vi "Shooter Immediate.vi"(7 "Description":string, 8 "Command Info In":T1, 9 "Deadband Value":dbl=0.01, 10 "LimeLightDistance?":bool, 11 "Setpoint":dbl) -> (0 "Command Info Out":T1)   [LabVIEW 2019]
doc: "This template includes code for deadband comparision to avoid excessive command scheduling. It is particularly useful for joystick-driven commands.\n\nBe sure to right-click and select New from Template and save with a new command name."
uses:
  <vilib>/Rock Robotics/WPI/Framework/Command Status Info.ctl
  <vilib>/Rock Robotics/WPI/Framework/Completion Status.ctl
  <vilib>/Rock Robotics/WPI/Framework/Completion Notifier.ctl
  Implementation/Shooter Setpoints.ctl
  Implementation/Shooter Operations.ctl
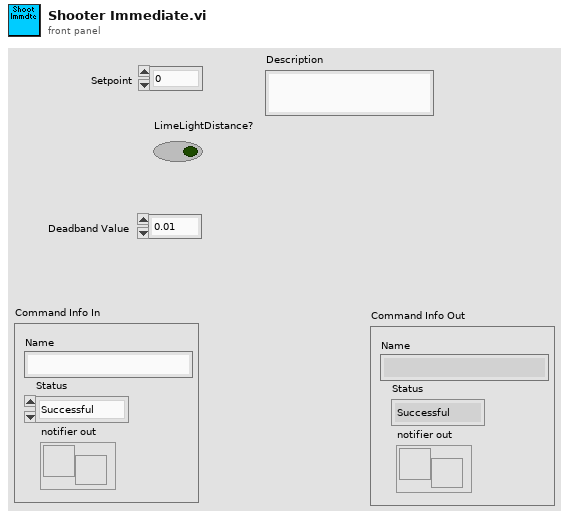
[diagram p1: front panel]
types:
  T1 = typedef "Command Status Info.ctl" = cluster{"Name":string, "Status":T2, "notifier out":T3}
  T2 = typedef "Completion Status.ctl" = enum16{"Successful", "Aborted", "Incomplete"}
  T3 = typedef "Completion Notifier.ctl" = refnum<notifier>
  T4 = typedef "Shooter Setpoints.ctl" = cluster{"Operation":T5, "Setpoint":dbl, "Duration":dbl, "LimelightSpeed":bool}
  T5 = typedef "Shooter Operations.ctl" = enum16{"Reserve", "Read Current", "Immediate", "Shoot for Time"}
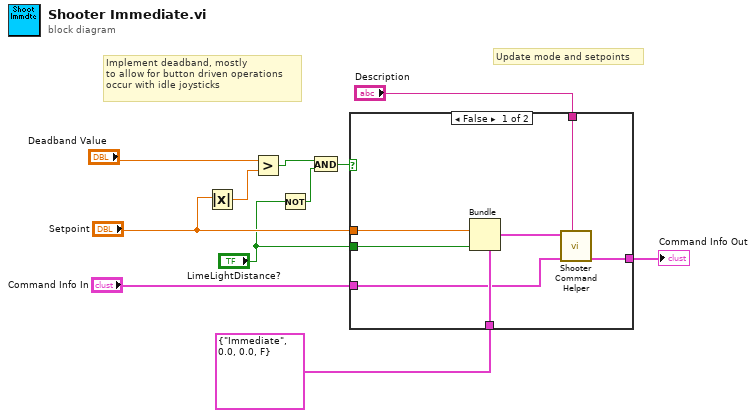
[diagram p0: block diagram]
diagram:
  # "Implement deadband, mostly\nto allow for button driven operations\noccur with idle joysticks"
  # "Update mode and setpoints"
  n1 = Absolute Value(x="Setpoint") -> (abs(x)=w10:dbl)
  n2 = Greater?(x="Deadband Value", y=w10) -> (0:w2:bool)
  n3 = Not(x="LimeLightDistance?") -> (.not. x?=w3:bool)
  n4 = And(x=w2, y=w3) -> (x .and. y?=w4:bool)
  n5 = case shown="False" w4 {
    tunnel: "Setpoint" -> [w18 _]
    tunnel: T4 {"Operation"=enum."Immediate", "Setpoint"=0.0, "Duration"=0.0, "LimelightSpeed"=FALSE} ("SubSystem Data") -> [w17 _]
    tunnel: [w16 w19] -> w9
    tunnel: "Command Info In" -> [w15 w19]
    tunnel: "Description" -> [w13 _]
    tunnel: "LimeLightDistance?" -> [w12 _]
    frame False {
      n6 = Bundle(cluster=w17, "Setpoint"=w18, "LimelightSpeed"=w12) -> (w14:T4)  [unwired: 2 in]
      n7 = call "Shooter Command Helper.vi"("Description"=w13, "Command Info In"=w15, "SubSystem Data"=w14) -> ("Command Info Out"=w16:T1)  [unwired: 6 in, 2 out]
    }
    frame True {
    }
  }
  "Command Info Out" <- w9
